vi "Adapt Variant Data To Type.vi"(5 "Type and Defaults":variant, 7 "Nulls as Defaults?":bool, 8 "error in (no error)":errorcluster, 10 "Variant in":variant) -> (0 "error out":errorcluster, 2 "Variant out":variant)   [LabVIEW 2020, in "openg_variant.lvlib"]
uses:
  openg_variant.lvlib
  LabVIEW Object/Reflection/getObjectPrivateData.vi
  LabVIEW Object/Reflection/extractObjectPrivateDataValues.vi
  <vilib>/Utility/LVClass/Get LV Class Name.vi
  LabVIEW Object/Reflection/reflectionPool.vi
  Array of VData to VCluster.vi
  <vilib>/Utility/Data Type/NI_Data Type.lvlib
panel:
  # "EXPERIMENTAL"
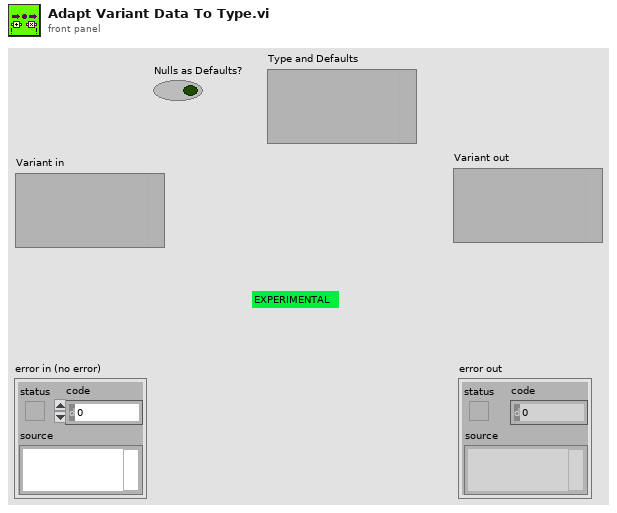
[diagram p1: front panel]
types:
  T1 = typedef "NI_Data Type.lvlib/Data Type.ctl" = enum8{"Invalid Type", "Void", "I8", "I16", "I32", "I64", "U8", "U16", "U32", "U64", "Single Float", "Double Float", "Extended Float", "Single Complex", "Double Complex", "Extended Complex", "Enum U8", "Enum U16", "Enum U32", "Enum U64", "Single Float With Unit", "Double Float With Unit", "Extended Float With Unit", "Single Complex with Unit", "Double Complex with Unit", "Extended Complex with Unit", "Boolean", "String", "Path", "Picture", "Tag", "Array", "Cluster", "Variant", "LV Variant", "Waveform", "Timestamp", "Digital Waveform", "Digital Data", "ExpressData", "Refnum", "External Data", "VI", "Poly VI", "LabVIEW Class Instance", "Fixed Point", "Set Collection", "Map Collection"}
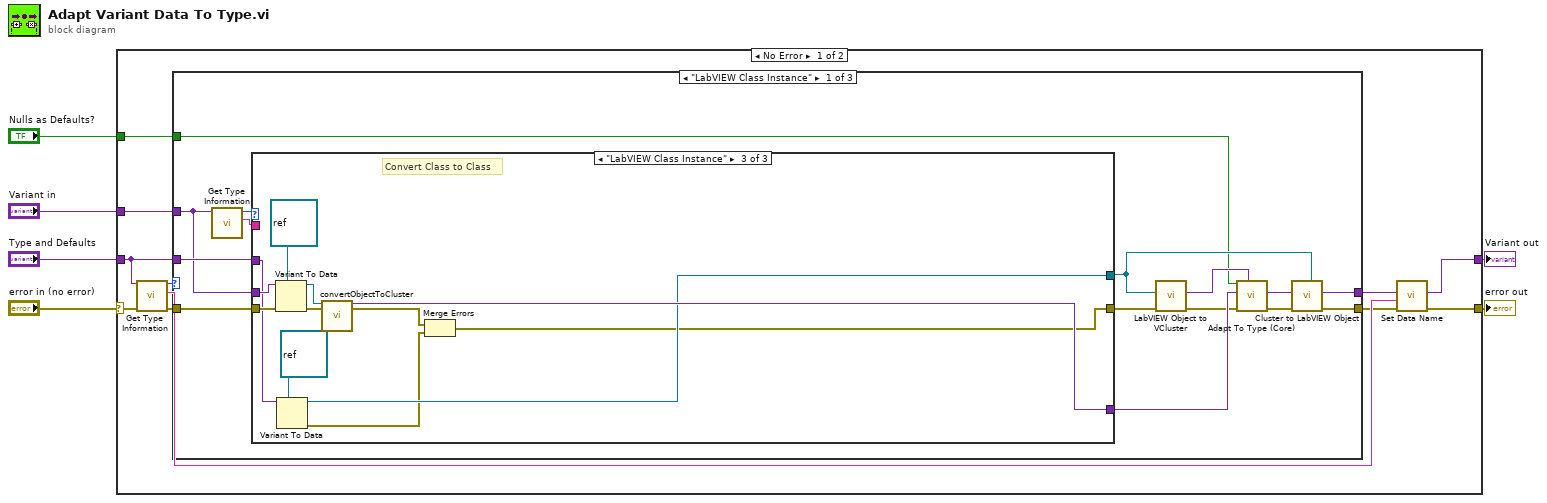
[diagram p0: block diagram]
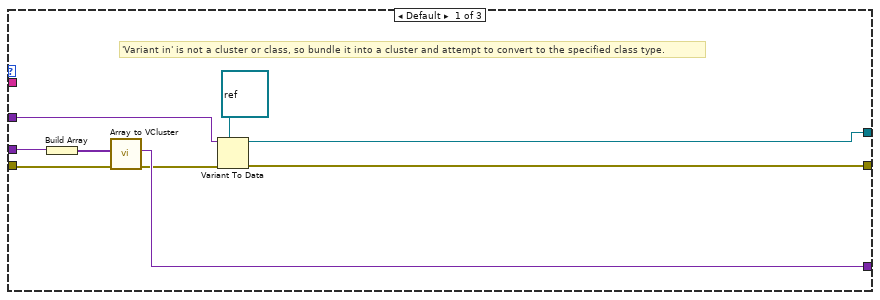
[diagram p2: hidden frame]
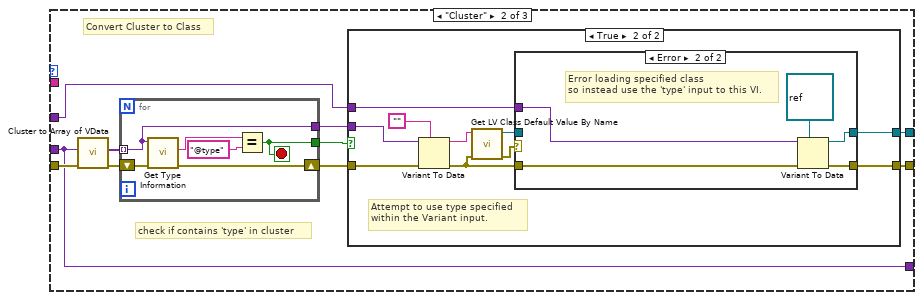
[diagram p3: hidden frame]
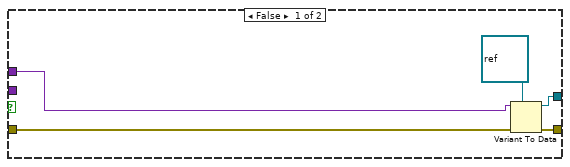
[diagram p4: hidden frame]
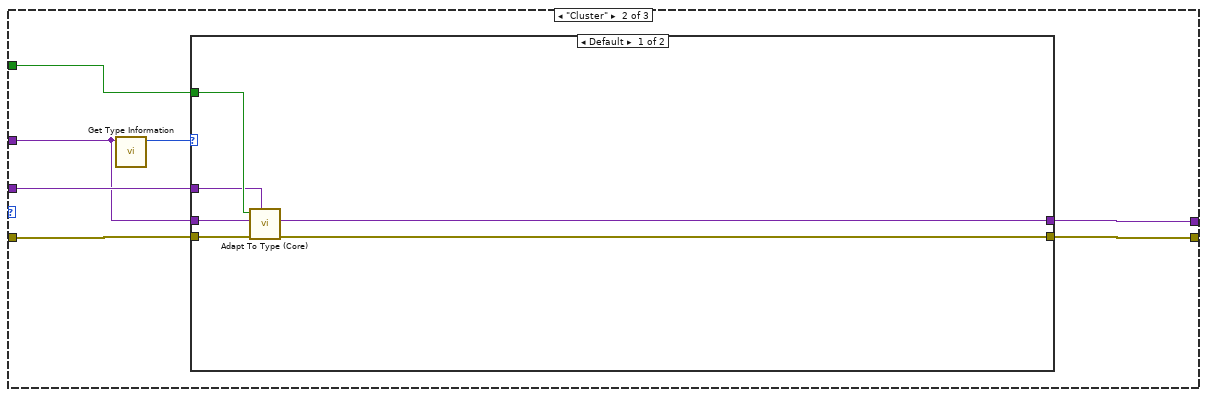
[diagram p6: hidden frame]
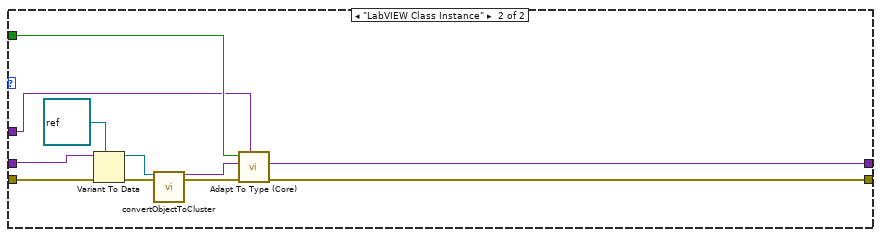
[diagram p7: hidden frame]
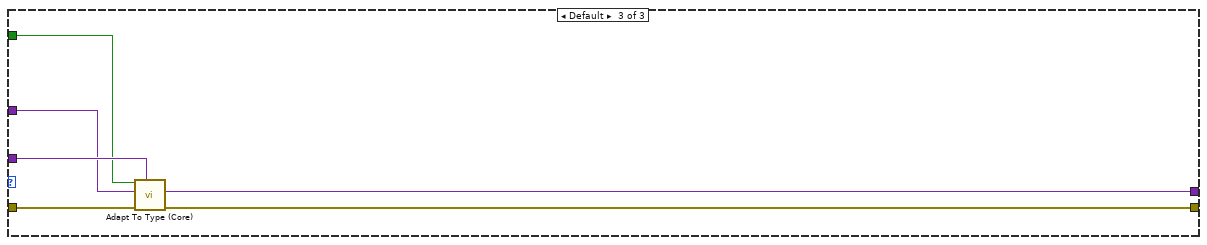
[diagram p8: hidden frame]
diagram:
  n1 = case shown="No Error" "error in (no error)" {
    selector: "error in (no error)" -> [w17 w122]
    tunnel: [w7 w122] -> w6
    tunnel: [w9 w123] -> w5
    tunnel: "Type and Defaults" -> [w13 w123]
    tunnel: "Variant in" -> [w12 _]
    tunnel: "Nulls as Defaults?" -> [w16 _]
    frame No Error {
      n2 = call <vilib>:"Get Type Information.vi"("error in (no error)"=w17, "variant"=w13) -> ("error out"=w15:errorcluster, "name"=w10:string, "type"=w14:T1)  [unwired: 5 in, 2 out]
      n3 = case shown="\"LabVIEW Class Instance\"" w14 {
        tunnel: [w32 w93 w121] -> w8
        tunnel: [w31 w92 w120] -> w11
        tunnel: w13 -> [w27 w96 w119]
        tunnel: w16 -> [w22 w97 w118]
        tunnel: w15 -> [w29 w94 w117]
        tunnel: w12 -> [w25 w95 w116]
        frame "LabVIEW Class Instance" {
          n4 = call <vilib>:"Get Type Information.vi"("variant"=w25) -> ("name"=w24:string, "type"=w26:T1)  [unwired: 6 in, 3 out]
          n5 = case shown="\"LabVIEW Class Instance\"" w26 {
            tunnel: [w33 w51 w82] -> w30
            tunnel: w29 -> [w38 w48 w87]
            tunnel: [w34 w45 w80] -> w28
            tunnel: w27 -> [w36 w44 w86]
            tunnel: w25 -> [w40 w42 w88]
            tunnel: [w39 w42 w84] -> w21
            tunnel: w24 -> [_ _ _]
            frame Default {
              # "'Variant in' is not a cluster or class, so bundle it into a cluster and attempt to convert to the specified class type."
              n6 = Build Array(w40) -> (w41:variant[])
              n7 = call "Array to VCluster.vi"("error in (no error)"=w38, "Array"=w41) -> ("error out"=w35:errorcluster, "VCluster"=w39:variant)  [unwired: 8 in]
              n8 = Variant To Data(error in=w35, type=refnum<class> refnum ("LabVIEW Object"), Variant=w36) -> (data=w33:refnum<class>, error out=w34:errorcluster)
            }
            frame "Cluster" {
              # "check if contains 'type' in cluster"
              # "Convert Cluster to Class"
              n9 = call "Cluster to Array of VData.vi"("error in (no error)"=w48, "Cluster"=w42) -> ("error out"=w47:errorcluster, "Array of VData"=w49:variant[])  [unwired: 8 in]
              n10 = for {
                tunnel: w49 -> [w52] mode=indexing
                shift-right: [w56] -> w43
                shift-left: w47 -> [w57]
                tunnel: [w53] -> w50
                tunnel: [w52] -> w46
                stop <- w53 stop-if-true
                n11 = call <vilib>:"Get Type Information.vi"("error in (no error)"=w57, "variant"=w52) -> ("error out"=w56:errorcluster, "name"=w55:string)  [unwired: 5 in, 3 out]
                n12 = Equal?(x=w55, y="@type") -> (x = y?=w53:bool)
              }
              n13 = case shown="True" w50 {
                tunnel: [w58 w71] -> w51
                tunnel: w46 -> [_ w68]
                tunnel: w43 -> [w60 w69]
                tunnel: [w59 w65] -> w45
                tunnel: w44 -> [w62 w63]
                frame False {
                  n14 = Variant To Data(error in=w60, type=refnum<class> refnum ("LabVIEW Object"), Variant=w62) -> (data=w58:refnum<class>, error out=w59:errorcluster)
                }
                frame True {
                  # "Attempt to use type specified\nwithin the Variant input."
                  n15 = Variant To Data(error in=w69, type="", Variant=w68) -> (data=w67:string, error out=w64:errorcluster)
                  n16 = call <vilib>:"Get LV Class Default Value By Name.vi"("error in (no error)"=w64, "class name"=w67) -> ("error out"=w66:errorcluster, "object"=w72:refnum<class>)  [unwired: 8 in]
                  n17 = case shown="Error" w66 {
                    tunnel: w72 -> [w74 _]
                    tunnel: [w74 w77] -> w71
                    tunnel: [w73 w75] -> w65
                    tunnel: w64 -> [w73 w76]
                    tunnel: w63 -> [_ w78]
                    frame No Error {
                    }
                    frame Error {
                      # "Error loading specified class\nso instead use the 'type' input to this VI."
                      n18 = Variant To Data(error in=w76, type=refnum<class> refnum ("LabVIEW Object"), Variant=w78) -> (data=w77:refnum<class>, error out=w75:errorcluster)
                    }
                  }
                }
              }
            }
            frame "LabVIEW Class Instance" {
              # "Convert Class to Class"
              n19 = Variant To Data(error in=w87, type=refnum<class> refnum ("LabVIEW Object"), Variant=w88) -> (data=w90:refnum<class>, error out=w91:errorcluster)
              n20 = Variant To Data(type=refnum<class> refnum ("LabVIEW Object"), Variant=w86) -> (data=w82:refnum<class>, error out=w81:errorcluster)  [unwired: 1 in]
              n21 = call "convertObjectToCluster.vi"("LabVIEW Object in"=w90, "error in (no error)"=w91) -> ("VCluster"=w84:variant, "error out"=w83:errorcluster)  [unwired: 16 in]
              n22 = Merge Errors(w83, w81) -> (w80:errorcluster)
            }
          }
          n23 = call "LabVIEW Object to VCluster.vi"("error in (no error)"=w28, "LabVIEW Object"=w30) -> ("error out"=w20:errorcluster, "VCluster"=w23:variant)  [unwired: 8 in]
          n24 = call "Adapt To Type (Core).vi"("Type and Defaults"=w23, "error in (no error)"=w20, "Variant in"=w21, "Nulls as Defaults?"=w22) -> ("error out"=w18:errorcluster, "Variant out"=w19:variant)  [unwired: 6 in]
          n25 = call "Cluster to LabVIEW Object.vi"("VObject Type"=w30, "error in (no error)"=w18, "VCluster"=w19) -> ("error out"=w32:errorcluster, "VObject out"=w31:variant)  [unwired: 7 in]
        }
        frame "Cluster" {
          n26 = call <vilib>:"Get Type Information.vi"("variant"=w95) -> ("type"=w98:T1)  [unwired: 6 in, 4 out]
          n27 = case shown="Default" w98 {
            tunnel: w97 -> [w104 w109]
            tunnel: w96 -> [w103 w108]
            tunnel: w95 -> [w102 w113]
            tunnel: w94 -> [w101 w114]
            tunnel: [w100 w106] -> w93
            tunnel: [w99 w105] -> w92
            frame Default {
              n28 = call "Adapt To Type (Core).vi"("Type and Defaults"=w103, "error in (no error)"=w101, "Variant in"=w102, "Nulls as Defaults?"=w104) -> ("error out"=w100:errorcluster, "Variant out"=w99:variant)  [unwired: 6 in]
            }
            frame "LabVIEW Class Instance" {
              n29 = Variant To Data(error in=w114, type=refnum<class> refnum ("objectType"), Variant=w113) -> (data=w112:refnum<class>, error out=w111:errorcluster)
              n30 = call "convertObjectToCluster.vi"("LabVIEW Object in"=w112, "error in (no error)"=w111) -> ("VCluster"=w110:variant, "error out"=w107:errorcluster)  [unwired: 16 in]
              n31 = call "Adapt To Type (Core).vi"("Type and Defaults"=w108, "error in (no error)"=w107, "Variant in"=w110, "Nulls as Defaults?"=w109) -> ("error out"=w106:errorcluster, "Variant out"=w105:variant)  [unwired: 6 in]
            }
          }
        }
        frame Default {
          n32 = call "Adapt To Type (Core).vi"("Type and Defaults"=w119, "error in (no error)"=w117, "Variant in"=w116, "Nulls as Defaults?"=w118) -> ("error out"=w121:errorcluster, "Variant out"=w120:variant)  [unwired: 6 in]
        }
      }
      n33 = call "Set Data Name.vi"("error in (no error)"=w8, "Data Name"=w10, "Data"=w11) -> ("error out"=w7:errorcluster, "Renamed Data"=w9:variant)  [unwired: 7 in]
    }
    frame Error {
    }
  }
  "error out" <- w6
  "Variant out" <- w5
